vi "Read Value (Signaling).vi"(8 "error in (no error)":errorcluster, 11 "DoValueSignal in":refnum<class "DoValueSignal.lvclass">) -> (0 "error out":errorcluster, 2 "Value (Signaling)":variant, 3 "DoValueSignal out":refnum<class "DoValueSignal.lvclass">)   [LabVIEW 2016, in "DoValueSignal.lvclass"]
uses:
  DoValueSignal.lvclass
  DoValueSignal.lvclass/DoValueSignal.ctl
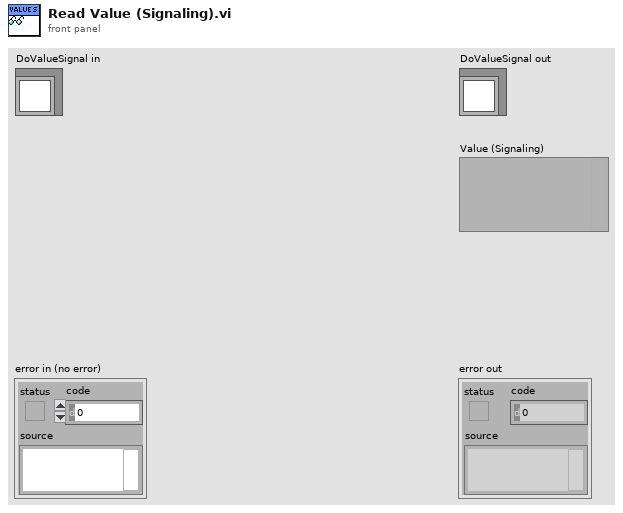
[diagram p1: front panel]
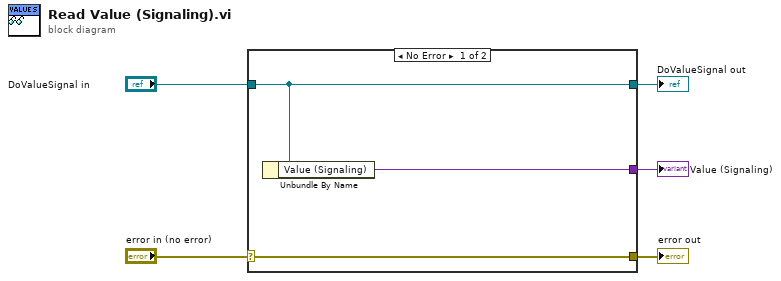
[diagram p0: block diagram]
diagram:
  n1 = case shown="No Error" "error in (no error)" {
    selector: "error in (no error)" -> [w8 w9]
    tunnel: [w8 w9] -> w4
    tunnel: [w7 w10] -> w2
    tunnel: "DoValueSignal in" -> [w7 w10]
    tunnel: [w6 _] -> w1
    frame No Error {
      n2 = Unbundle By Name(w7) -> ("Value (Signaling)"=w6:variant)
    }
    frame Error {
    }
  }
  "error out" <- w4
  "DoValueSignal out" <- w2
  "Value (Signaling)" <- w1
